vi "PLC_Decode (SubVI).vi"(10 "Coils read":map{string, bool}(c390), 11 "Values read":map{string, dbl}(c390)) -> (2 "Coils read out":map{string, bool}(c390), 3 "Values read out":map{string, dbl}(c390))   [LabVIEW 2024]
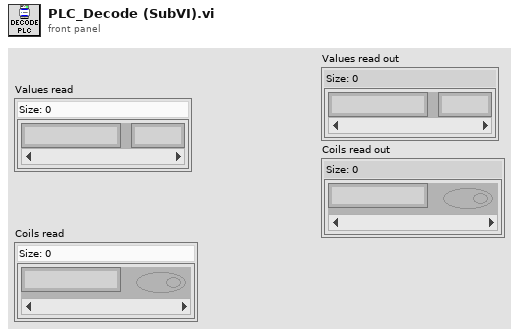
[diagram p1: front panel]
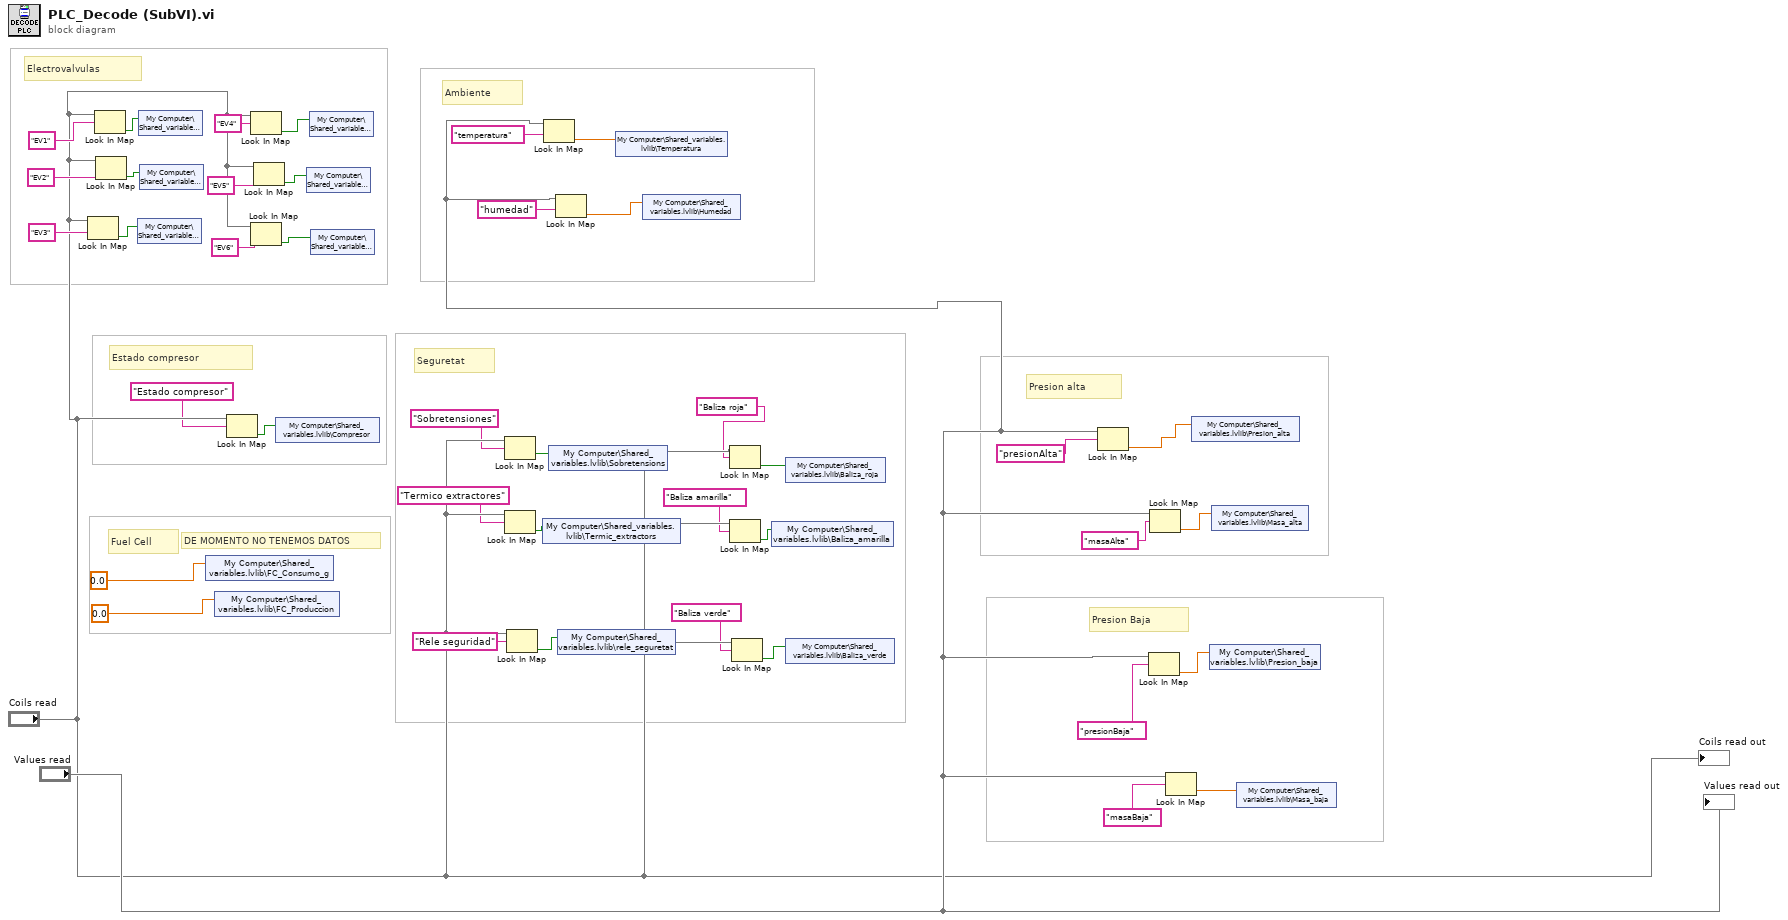
[diagram p0: block diagram]
diagram:
  # "Electrovalvulas"
  # "Ambiente"
  # "Seguretat"
  # "Presion Baja"
  # "Presion alta"
  # "DE MOMENTO NO TENEMOS DATOS"
  # "Fuel Cell"
  # "Estado compresor"
  n1 = Look In Map(map="Coils read", key="EV3") -> (value=w22:bool)  [unwired: 1 in, 1 out]
  n2 = Look In Map(map="Coils read", key="EV1") -> (value=w24:bool)  [unwired: 1 in, 1 out]
  n3 = Look In Map(map="Coils read", key="EV2") -> (value=w23:bool)  [unwired: 1 in, 1 out]
  n4 = shared-variable "My Computer\\Shared_variables.lvlib\\EV3"(w22) -> ()  [unwired: 1 in, 1 out]
  n5 = shared-variable "My Computer\\Shared_variables.lvlib\\EV1"(w24) -> ()  [unwired: 1 in, 1 out]
  n6 = shared-variable "My Computer\\Shared_variables.lvlib\\EV2"(w23) -> ()  [unwired: 1 in, 1 out]
  n7 = shared-variable "My Computer\\Shared_variables.lvlib\\FC_Consumo_g"(0.0 ("g H2 consumidos por la FC")) -> ()  [unwired: 1 in, 1 out]
  n8 = shared-variable "My Computer\\Shared_variables.lvlib\\FC_Produccion"(0.0 ("Producción FC")) -> ()  [unwired: 1 in, 1 out]
  n9 = Look In Map(map="Coils read", key="Estado compresor") -> (value=w30:bool)  [unwired: 1 in, 1 out]
  n10 = Look In Map(map="Coils read", key="EV4") -> (value=w27:bool)  [unwired: 1 in, 1 out]
  n11 = Look In Map(map="Coils read", key="EV6") -> (value=w25:bool)  [unwired: 1 in, 1 out]
  n12 = Look In Map(map="Coils read", key="EV5") -> (value=w26:bool)  [unwired: 1 in, 1 out]
  n13 = shared-variable "My Computer\\Shared_variables.lvlib\\Compresor"(w30) -> ()  [unwired: 1 in, 1 out]
  n14 = shared-variable "My Computer\\Shared_variables.lvlib\\EV5"(w26) -> ()  [unwired: 1 in, 1 out]
  n15 = shared-variable "My Computer\\Shared_variables.lvlib\\EV4"(w27) -> ()  [unwired: 1 in, 1 out]
  n16 = shared-variable "My Computer\\Shared_variables.lvlib\\EV6"(w25) -> ()  [unwired: 1 in, 1 out]
  n17 = Look In Map(map="Coils read", key="Sobretensiones") -> (value=w40:bool)  [unwired: 1 in, 1 out]
  n18 = Look In Map(map="Coils read", key="Termico extractores") -> (value=w41:bool)  [unwired: 1 in, 1 out]
  n19 = Look In Map(map="Coils read", key="Rele seguridad") -> (value=w42:bool)  [unwired: 1 in, 1 out]
  n20 = shared-variable "My Computer\\Shared_variables.lvlib\\Termic_extractors"(w41) -> ()  [unwired: 1 in, 1 out]
  n21 = Look In Map(map="Values read", key="temperatura") -> (value=w28:dbl)  [unwired: 1 in, 1 out]
  n22 = shared-variable "My Computer\\Shared_variables.lvlib\\Sobretensions"(w40) -> ()  [unwired: 1 in, 1 out]
  n23 = Look In Map(map="Values read", key="humedad") -> (value=w29:dbl)  [unwired: 1 in, 1 out]
  n24 = shared-variable "My Computer\\Shared_variables.lvlib\\rele_seguretat"(w42) -> ()  [unwired: 1 in, 1 out]
  n25 = shared-variable "My Computer\\Shared_variables.lvlib\\Temperatura"(w28) -> ()  [unwired: 1 in, 1 out]
  n26 = shared-variable "My Computer\\Shared_variables.lvlib\\Humedad"(w29) -> ()  [unwired: 1 in, 1 out]
  n27 = Look In Map(map="Coils read", key="Baliza roja") -> (value=w35:bool)  [unwired: 1 in, 1 out]
  n28 = Look In Map(map="Coils read", key="Baliza amarilla") -> (value=w34:bool)  [unwired: 1 in, 1 out]
  n29 = Look In Map(map="Coils read", key="Baliza verde") -> (value=w33:bool)  [unwired: 1 in, 1 out]
  n30 = shared-variable "My Computer\\Shared_variables.lvlib\\Baliza_amarilla"(w34) -> ()  [unwired: 1 in, 1 out]
  n31 = shared-variable "My Computer\\Shared_variables.lvlib\\Baliza_roja"(w35) -> ()  [unwired: 1 in, 1 out]
  n32 = shared-variable "My Computer\\Shared_variables.lvlib\\Baliza_verde"(w33) -> ()  [unwired: 1 in, 1 out]
  n33 = Look In Map(map="Values read", key="presionAlta") -> (value=w36:dbl)  [unwired: 1 in, 1 out]
  n34 = Look In Map(map="Values read", key="presionBaja") -> (value=w39:dbl)  [unwired: 1 in, 1 out]
  n35 = Look In Map(map="Values read", key="masaAlta") -> (value=w37:dbl)  [unwired: 1 in, 1 out]
  n36 = Look In Map(map="Values read", key="masaBaja") -> (value=w38:dbl)  [unwired: 1 in, 1 out]
  n37 = shared-variable "My Computer\\Shared_variables.lvlib\\Presion_alta"(w36) -> ()  [unwired: 1 in, 1 out]
  n38 = shared-variable "My Computer\\Shared_variables.lvlib\\Presion_baja"(w39) -> ()  [unwired: 1 in, 1 out]
  n39 = shared-variable "My Computer\\Shared_variables.lvlib\\Masa_alta"(w37) -> ()  [unwired: 1 in, 1 out]
  n40 = shared-variable "My Computer\\Shared_variables.lvlib\\Masa_baja"(w38) -> ()  [unwired: 1 in, 1 out]
  "Values read out" <- "Values read"
  "Coils read out" <- "Coils read"
